vi "DAQ_Ejemplo02.vi"() -> ()   [LabVIEW 2020]
panel:
  out "XY Graph 2":cluster{dbl[], dbl[]}(graph)
  out "XY Graph":cluster{dbl[], dbl[]}(graph)
  out "Waveform Chart":dynamicdata(graph)
  out "appended array 2":dbl[](array[numeric])
  out "appended array":dbl[](array[numeric])
  out "Waveform Graph":dynamicdata(graph)
  in  "stop":bool
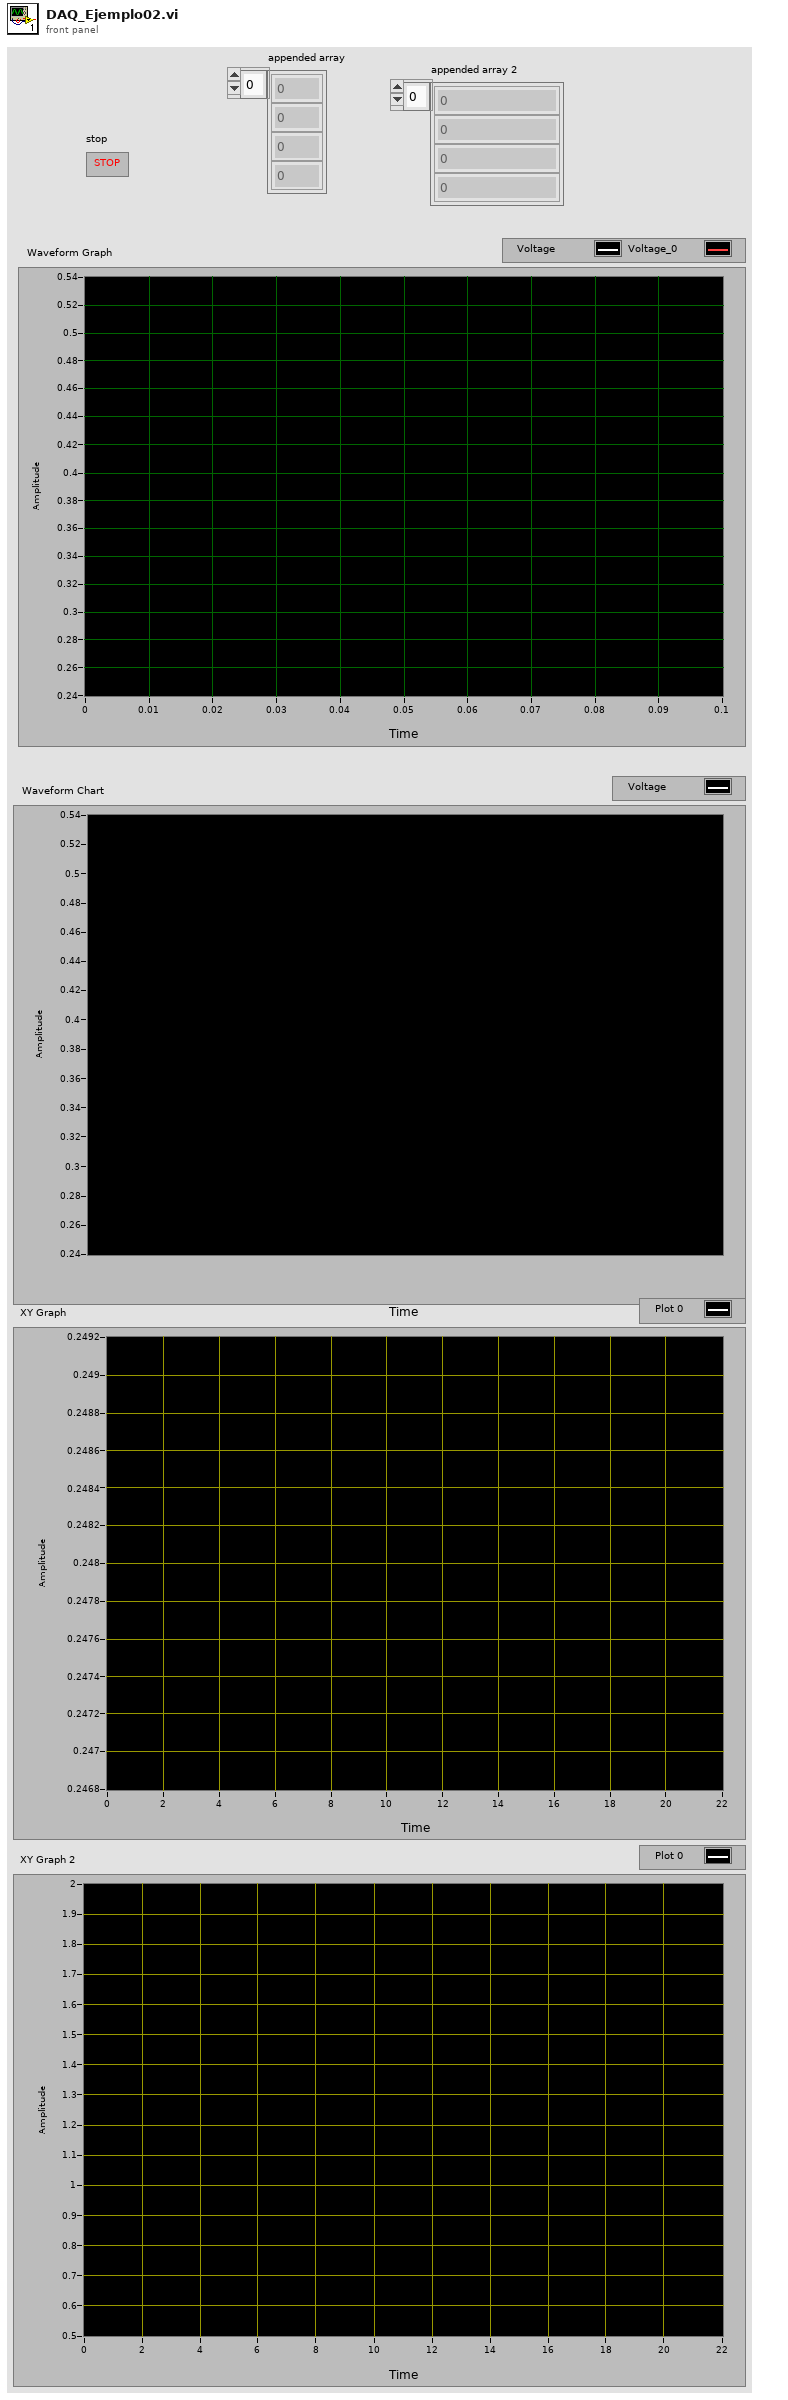
[diagram p1: front panel]
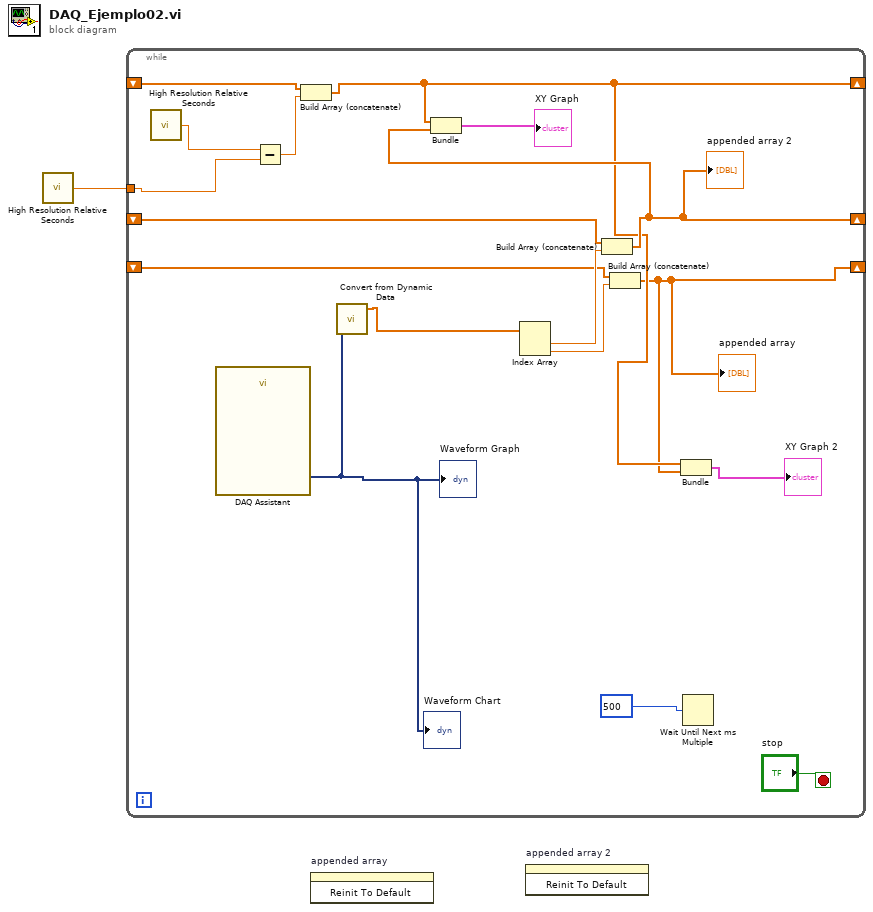
[diagram p0: block diagram]
diagram:
  n1 = call <vilib>:"High Resolution Relative Seconds.vi"() -> ("relative seconds"=w1:dbl)
  n2 = while {
    shift-right: [w3] -> _
    shift-left: _ -> [w13]
    shift-right: [w6] -> _
    shift-left: _ -> [w14]
    tunnel: w1 -> [w9]
    shift-right: [w4] -> _
    shift-left: _ -> [w7]
    stop <- "stop" stop-if-true
    n3 = call <vilib>:"High Resolution Relative Seconds.vi"() -> ("relative seconds"=w10:dbl)
    n4 = call "DAQ Assistant"() -> ("data"=w11:dynamicdata)  [unwired: 17 in, 2 out]
    "Waveform Graph" <- w11
    "Waveform Chart" <- w11
    n5 = Subtract(x=w10, y=w9) -> (x-y=w8:dbl)
    n6 = Build Array (concatenate)(w7, w8) -> (w4:dbl[])
    n7 = call "Convert from Dynamic Data"("Dynamic Data Type"=w11) -> ("Array"=w17:dbl[])  [unwired: 3 in]
    n8 = Index Array "Index Array"(array=w17) -> (element #1=w15:dbl, element #2=w16:dbl)  [unwired: 2 in]
    n9 = Build Array (concatenate)(w14, w15) -> (w6:dbl[])
    "appended array 2" <- w6
    n10 = Bundle(w4, w6) -> (→"XY Graph":cluster{dbl[], dbl[]})  [unwired: 1 in]
    n11 = Build Array (concatenate) "Build Array"(w13, w16) -> (w3:dbl[])
    "appended array" <- w3
    n12 = Bundle(w4, w3) -> (→"XY Graph 2":cluster{dbl[], dbl[]})  [unwired: 1 in]
    n13 = Wait Until Next ms Multiple(millisecond multiple=u32 500 ("milliseconds to wait")) -> ()  [unwired: 1 out]
  }
  n14 = invoke on="appended array" class="Arr (strict)" method="Reinit To Default"() -> ()  [unwired: 3 in, 3 out]
  n15 = invoke on="appended array 2" class="Arr (strict)" method="Reinit To Default"() -> ()  [unwired: 3 in, 3 out]
